vi "EXAMPLE64.VI"() -> ()   [LabVIEW 2014]
uses:
  wlcomp.dll
  C:/Program Files (x86)/LCard/LIBRARY/BIN/wlcomp64.dll
panel:
  out "Numeric":i32
  out "Краткое описание":string="Данный пример поддерживает платы L761 L780 L783 L791 и модули E-154 E14-140 E14-440 E20-10. В примере осуществляется сбор 8192 отсчетов с 4 каналов АЦП на максимальной скорости (для E20-10 на скорости 1МГц). Перед началом работы необходимо ввести имя фала с биос для платы (без расширения, для модулей без биоса произвольно) и номер слота, где установлена плата. См. также файд instruct.html."
  out "TTL Input (IoAsync demo)":i32
  in  "SynchroType\n3 - without sync(L7XX E2010)\n0 - without sync(E440 E140 E154 L791)":u32=3
  in  "Enter slot number":u32
  in  "Enter bios name":string="l761"
  out "Display":i16[][](graph)
  out "sync counter":u32
  in  "stop":bool
  out "data addr":u32
  out "sync addr":u32
  out "size":u32
  out "dRate":dbl format="%.2f"
  out "FIFO":u32
  out "IrqStep":u32
  out "Pages":u32
  out "Alloc":u32
  out "Error":u32
  out "IsDacPresent":u16
  out "Quartz":i32
  out "DspType":string
  out "Rev":string
  out "BrdName":string
  out "SerNum":string
  out "Base I/O":u32 format="%.0x"
  out "Irq":u32
  out "Dsp":u32
  out "BoardType":u32
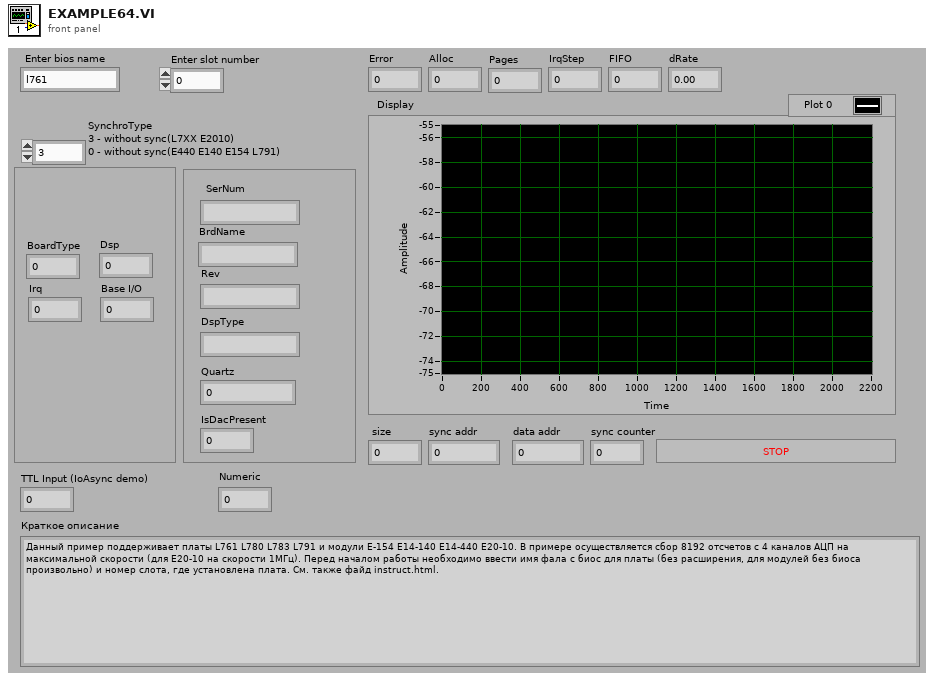
[diagram p1: front panel]
types:
  T1 = cluster{"s_Type":u32, "FIFO":u32, "IrqStep":u32, "Pages":u32, "Autoinit":u32, "dRate":dbl, "dKadr":dbl, "dScale":dbl, "Rate":u32, "Kadr":u32, "Scale":u32, "FPDelay":u32, "SynchroType\n3 - without sync(L7XX E2010)\n0 - without sync(E440 E140 E154 L791)":u32, "SynchroSensitivity":u32, "SynchroMode":u32, "AdChannel":u32, "AdPorog":u32, "NCh":u32, u32[], "IrqEna":u32, "AdcEna":u32}
  T2 = cluster{"[0]":u32, "[1]":u32, "[2]":u32, "[3]":u32, "[4]":u32, "[5]":u32, "[6]":u32, "[7]":u32, "[8]":u32, "[9]":u32, "[10]":u32, "[11]":u32, "[12]":u32, "[13]":u32, "[14]":u32, "[15]":u32, "[16]":u32, "[17]":u32, "[18]":u32, "[19]":u32}
  T3 = cluster{string, string, string, string, i32, u16}
  T4 = cluster{"s_Type":u32, "FIFO":u32, "IrqStep":u32, "Pages":u32, "dRate":dbl, "Rate":u32, "NCh":u32, "Chn[0]":u32, "Data[0]":u32, "Chn[1]":u32, "Data[1]":u32, "Mode":u32}
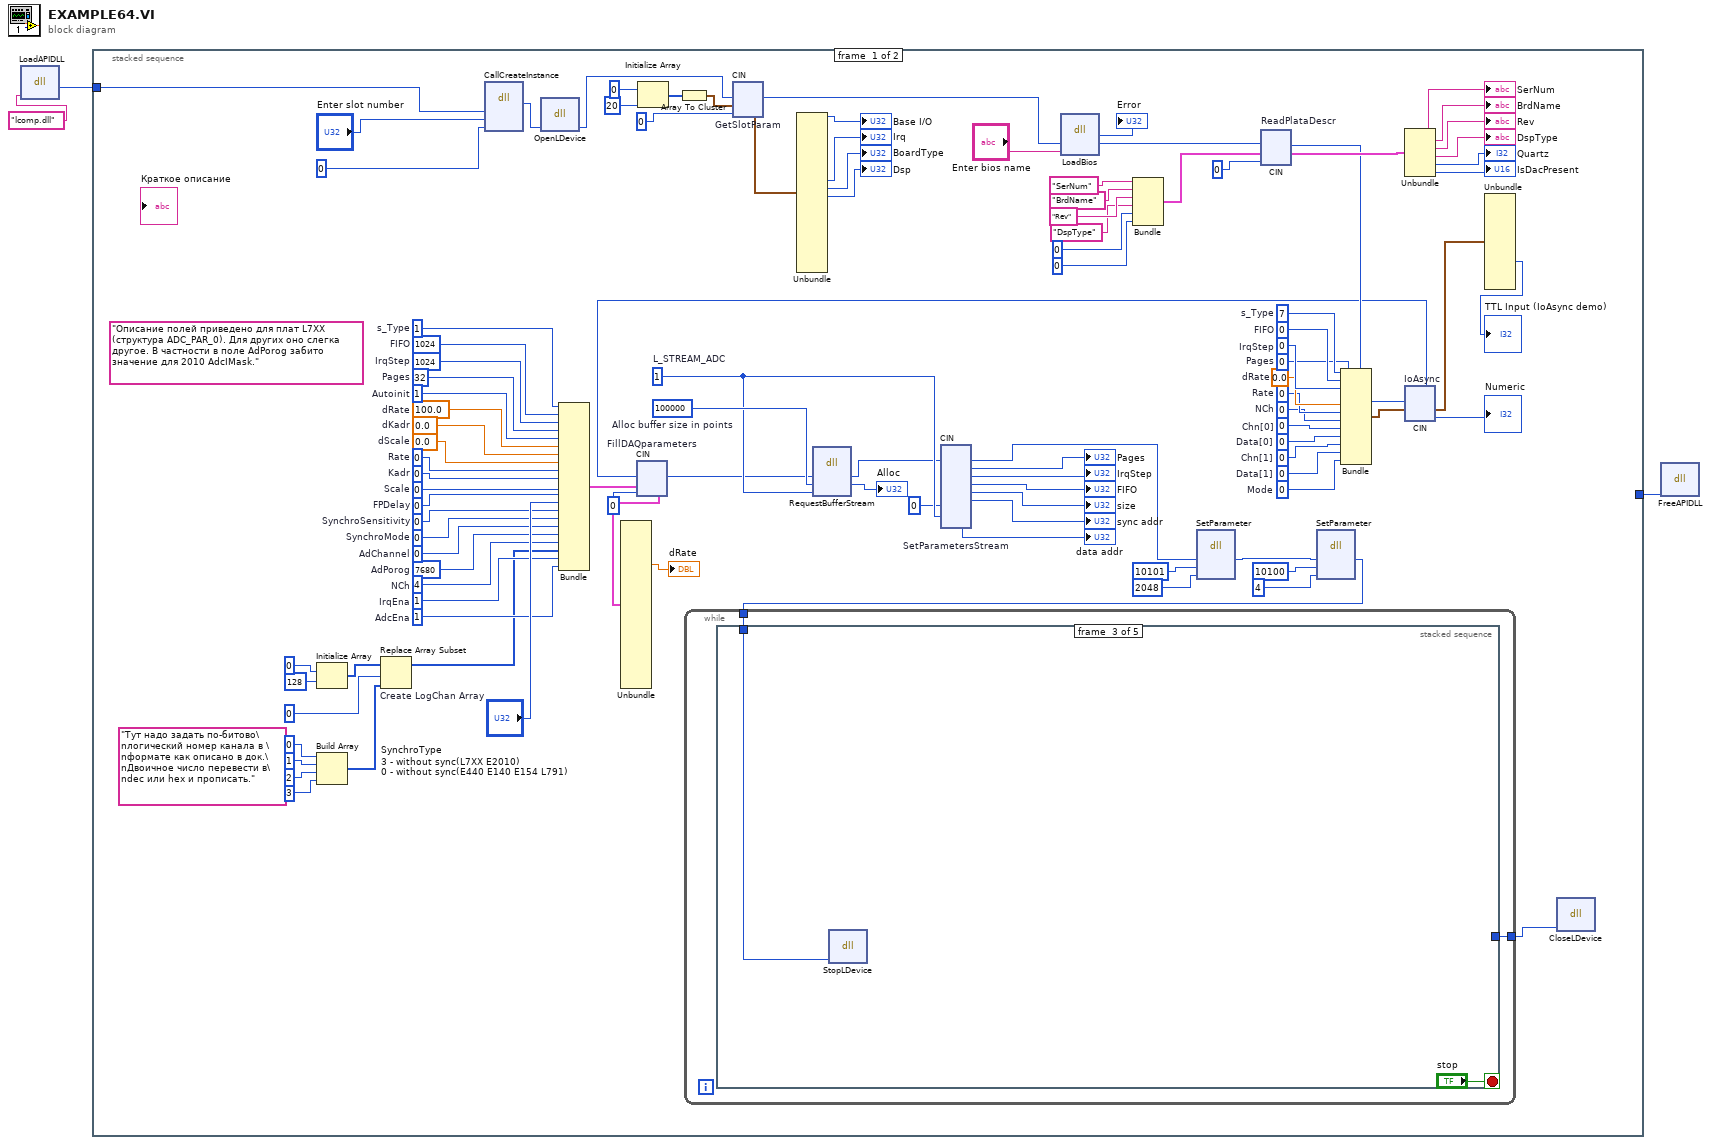
[diagram p0: block diagram]
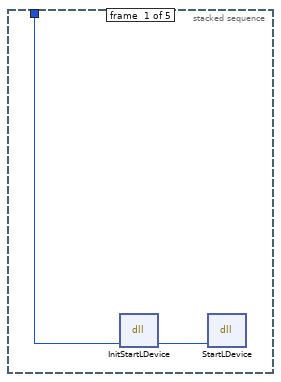
[diagram p2: hidden frame]
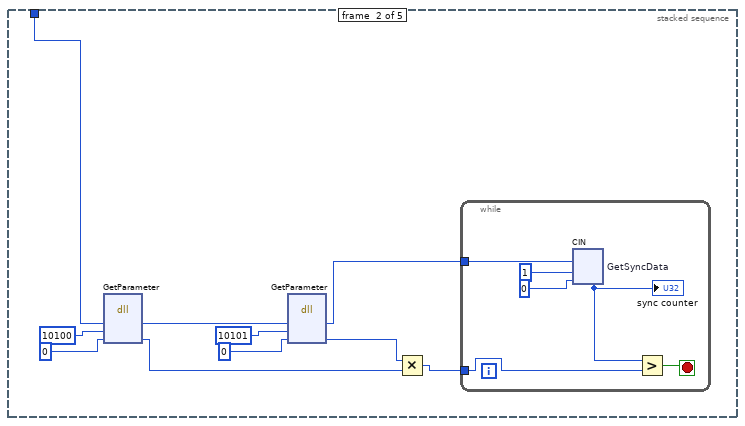
[diagram p3: hidden frame]
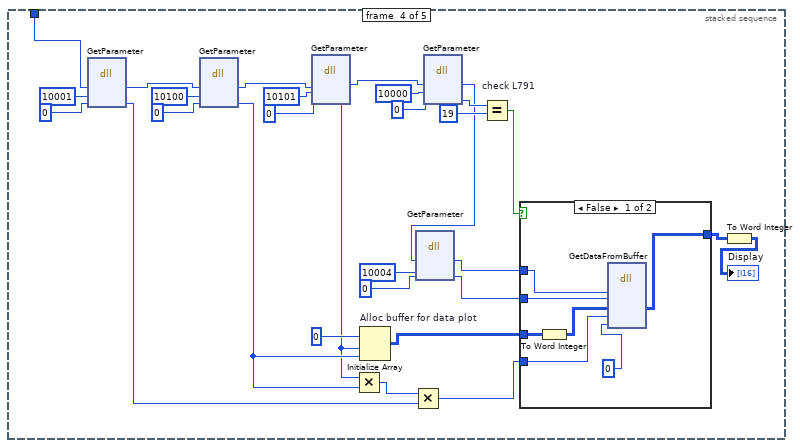
[diagram p4: hidden frame]
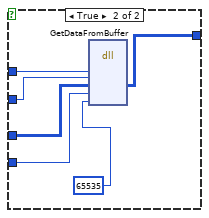
[diagram p5: hidden frame]
diagram:
  n1 = dll-call lib="wlcomp.dll" fn="LoadAPIDLL" label="LoadAPIDll"("dllname"="lcomp.dll") -> (w1:u32)  [unwired: 4 in, 2 out]
  n2 = stacked-sequence {
    tunnel: w1 -> [w105 w175]
    tunnel: [_ w175] -> w2
    frame #0 {
      w4 = u32 0  # Data[1]
      w5 = u32 0  # Chn[1]
      (unwired) "Тут надо задать по-битово\nлогический номер канала в \nформате как описано в док.\nДвоичное число перевести в\ndec или hex и прописать."
      (unwired) "Описание полей приведено для плат L7XX (структура ADC_PAR_0). Для других оно слегка другое. В частности в поле AdPorog забито значение для 2010 AdcIMask."
      w32 = u32 0  # Mode
      w23 = u32 0  # Data[0]
      w24 = u32 0  # Chn[0]
      w25 = u32 0  # NCh
      w26 = u32 0  # Rate
      w27 = 0.0  # dRate
      w28 = u32 0  # Pages
      w29 = u32 0  # IrqStep
      w30 = u32 0  # FIFO
      w31 = u32 7  # s_Type
      w52 = u32 1  # L_STREAM_ADC
      w53 = u32 100000  # Alloc buffer size in points
      w64 = u32 1  # AdcEna
      w65 = u32 1  # IrqEna
      w66 = u32 4  # NCh
      w67 = u32 7680  # AdPorog
      w68 = u32 0  # AdChannel
      w69 = u32 0  # SynchroMode
      w70 = u32 0  # SynchroSensitivity
      w72 = u32 0  # FPDelay
      w73 = u32 0  # Scale
      w74 = u32 0  # Kadr
      w75 = u32 0  # Rate
      w76 = 0.0  # dScale
      w77 = 0.0  # dKadr
      w78 = 100.0  # dRate
      w79 = u32 1  # Autoinit
      w80 = u32 32  # Pages
      w81 = u32 1024  # IrqStep
      w82 = u32 1024  # FIFO
      w83 = u32 1  # s_Type
      n3 = Initialize Array(u32 0, u32 128) -> (w61:u32[])
      n4 = Build Array(0, 1, 2, 3) -> (w58:i32[])
      n5 = Replace Array Subset "Create LogChan Array"(array=w61, new element=w58, index=u32 0) -> (w60:u32[])
      n6 = dll-call lib="wlcomp.dll" fn="CallCreateInstance"("hDll"=w105, "slot"="Enter slot number", "Err"=u32 0) -> (w46:u32)  [unwired: 6 in, 2 out]
      n7 = dll-call lib="wlcomp.dll" fn="OpenLDevice"("hIfc"=w46) -> ("hIfc"=w45:u32)  [unwired: 4 in, 2 out]
      n8 = Bundle("s_Type"=w83, "FIFO"=w82, "IrqStep"=w81, "Pages"=w80, "Autoinit"=w79, "dRate"=w78, "dKadr"=w77, "dScale"=w76, "Rate"=w75, "Kadr"=w74, "Scale"=w73, "FPDelay"=w72, "SynchroType\n3 - without sync(L7XX E2010)\n0 - without sync(E440 E140 E154 L791)"="SynchroType\n3 - without sync(L7XX E2010)\n0 - without sync(E440 E140 E154 L791)", "SynchroSensitivity"=w70, "SynchroMode"=w69, "AdChannel"=w68, "AdPorog"=w67, "NCh"=w66, w60, "IrqEna"=w65, "AdcEna"=w64) -> (w84:T1)  [unwired: 1 in]
      n9 = Initialize Array(u32 0, u32 20) -> (w107:u32[])
      n10 = Array To Cluster(array=w107) -> (cluster=w99:T2)
      n11 = cin "GetSlotParam"(w45, w99, u32 0) -> (w39:u32, w98:T2)  [unwired: 1 in]
      n12 = Unbundle(w98) -> ("[0]"=→"Base I/O":u32, "[8]"=→"Irq":u32, "[9]"=→"BoardType":u32, "[10]"=→"Dsp":u32)  [unwired: 16 out]
      n13 = dll-call lib="wlcomp.dll" fn="LoadBios"("hIfc"=w39, "BiosName"="Enter bios name") -> (→"Error":u32, "hIfc"=w38:u32)  [unwired: 4 in, 2 out]
      n14 = Bundle("SerNum", "BrdName", "Rev", "DspType", 0, u16 0) -> (w35:T3)  [unwired: 1 in]
      n15 = cin "ReadPlataDescr"(w38, w35, u32 0) -> (w17:u32, w91:T3)  [unwired: 1 in]
      n16 = Bundle("s_Type"=w31, "FIFO"=w30, "IrqStep"=w29, "Pages"=w28, "dRate"=w27, "Rate"=w26, "NCh"=w25, "Chn[0]"=w24, "Data[0]"=w23, "Chn[1]"=w5, "Data[1]"=w4, "Mode"=w32) -> (w22:T4)  [unwired: 1 in]
      n17 = Unbundle(w91) -> (→"SerNum":string, →"BrdName":string, →"Rev":string, →"DspType":string, →"Quartz":i32, →"IsDacPresent":u16)
      n18 = cin "IoAsync"(w17, w22) -> (w16:u32, w21:T4, →"Numeric":i32)  [unwired: 1 in]
      n19 = cin "FillDAQparameters"(w16, w84, 0) -> (w42:u32, w34:T1)  [unwired: 1 in]
      n20 = Unbundle(w34) -> ("dRate"=→"dRate":dbl)  [unwired: 20 out]
      n21 = dll-call lib="wlcomp.dll" fn="RequestBufferStream" label="RequestBuffer"("hIfc"=w42, "Size"=w53, "StreamId"=w52) -> ("hIfc"=w41:u32, "Size"=→"Alloc":u32)  [unwired: 5 in, 2 out]
      n22 = cin "SetParametersStream"(w41, w52, u32 0) -> (w10:u32, →"Pages":u32, →"IrqStep":u32, →"FIFO":u32, →"size":u32, →"sync addr":u32, →"data addr":u32)  [unwired: 8 in]
      n23 = dll-call lib="wlcomp.dll" fn="SetParameter" label="Store point per chan"("hIfc"=w10, "name"=10101, "param"=2048) -> ("hIfc"=w6:u32)  [unwired: 6 in, 2 out]
      n24 = dll-call lib="wlcomp.dll" fn="SetParameter" label="Store NCh"("hIfc"=w6, "name"=10100, "param"=4) -> ("hIfc"=w7:u32)  [unwired: 6 in, 2 out]
      n25 = while {
        tunnel: w7 -> [w111]
        tunnel: [w110] -> w13
        stop <- "stop" stop-if-true
        n26 = stacked-sequence {
          tunnel: w111 -> [w113 w116 w131 w147 w174]
          tunnel: [_ _ _ _ w174] -> w110
          frame #0 {
            n27 = dll-call lib="wlcomp.dll" fn="InitStartLDevice"("hIfc"=w113) -> ("hIfc"=w114:u32)  [unwired: 4 in, 2 out]
            n28 = dll-call lib="wlcomp.dll" fn="StartLDevice"("hIfc"=w114) -> ()  [unwired: 5 in, 2 out]
          }
          frame #1 {
            n29 = dll-call lib="wlcomp.dll" fn="GetParameter" label="Get NCh"("hIfc"=w116, "name"=10100, "param"=0) -> ("hIfc"=w121:u32, "param"=w123:u32)  [unwired: 5 in, 2 out]
            n30 = dll-call lib="wlcomp.dll" fn="GetParameter" label="Get points per chan"("hIfc"=w121, "name"=10101, "param"=0) -> ("hIfc"=w115:u32, "param"=w122:u32)  [unwired: 5 in, 2 out]
            n31 = Multiply(x=w122, y=w123) -> (x*y=w124:u32)
            n32 = while {
              tunnel: w115 -> [w126]
              tunnel: w124 -> [w125]
              stop <- w130 stop-if-true
              n33 = cin "GetSyncData"(w126, 1, u32 0) -> (w127:u32)  [unwired: 2 in]
              "sync counter" <- w127
              n34 = Greater?(x=w127, y=w125) -> (0:w130:bool)
            }
          }
          frame #2 {
            n35 = dll-call lib="wlcomp.dll" fn="StopLDevice"("hIfc"=w131) -> ()  [unwired: 5 in, 2 out]
          }
          frame #3 {
            n36 = dll-call lib="wlcomp.dll" fn="GetParameter" label="Get DataPoint size"("hIfc"=w147, "name"=10001, "param"=0) -> ("hIfc"=w134:u32, "param"=w151:u32)  [unwired: 5 in, 2 out]
            n37 = dll-call lib="wlcomp.dll" fn="GetParameter" label="Get NCh"("hIfc"=w134, "name"=10100, "param"=0) -> ("hIfc"=w135:u32, "param"=w133:u32)  [unwired: 5 in, 2 out]
            n38 = dll-call lib="wlcomp.dll" fn="GetParameter" label="Get points per chan"("hIfc"=w135, "name"=10101, "param"=0) -> ("hIfc"=w138:u32, "param"=w132:u32)  [unwired: 5 in, 2 out]
            n39 = Multiply(x=w132, y=w133) -> (x*y=w146:u32)
            n40 = Initialize Array "Alloc buffer for data plot"(u32 0, w132, w133) -> (w154:u32[][])
            n41 = Multiply(x=w146, y=w151) -> (x*y=w156:u32)
            n42 = dll-call lib="wlcomp.dll" fn="GetParameter" label="Get BoardType"("hIfc"=w138, "name"=10000, "param"=0) -> ("hIfc"=w143:u32, "param"=w148:u32)  [unwired: 5 in, 2 out]
            n43 = dll-call lib="wlcomp.dll" fn="GetParameter" label="Get DataAddr"("hIfc"=w143, "name"=10004, "param"=0) -> ("hIfc"=w142:u32, "param"=w141:u32)  [unwired: 5 in, 2 out]
            n44 = Equal? "check L791"(x=w148, y=19) -> (x = y?=w159:bool)
            n45 = case shown="False" w159 {
              tunnel: [w167 w173] -> w158
              tunnel: w142 -> [w166 w172]
              tunnel: w141 -> [w165 w171]
              tunnel: w154 -> [w163 w170]
              tunnel: w156 -> [w164 w169]
              frame False {
                n46 = To Word Integer(number=w163) -> (16bit integer=w162:i16[][])
                n47 = dll-call lib="wlcomp.dll" fn="GetDataFromBuffer"("hIfc"=w166, "data"=w165, "datad"=w162, "size"=w164, "mask"=u32 0) -> ("datad"=w167:i16[][])  [unwired: 8 in, 2 out]
              }
              frame True {
                n48 = dll-call lib="wlcomp.dll" fn="GetDataFromBuffer"("hIfc"=w172, "data"=w171, "datad"=w170, "size"=w169, "mask"=65535) -> ("datad"=w173:u32[][])  [unwired: 8 in, 2 out]
              }
            }
            n49 = To Word Integer(number=w158) -> (16bit integer=→"Display":i16[][])
          }
          frame #4 {
          }
        }
      }
      n50 = Unbundle(w21) -> ("Data[0]"=→"TTL Input (IoAsync demo)":u32)  [unwired: 11 out]
      n51 = dll-call lib="wlcomp.dll" fn="CloseLDevice"("hIfc"=w13) -> ()  [unwired: 5 in, 2 out]
    }
    frame #1 {
    }
  }
  n52 = dll-call lib="C:/Program Files (x86)/LCard/LIBRARY/BIN/wlcomp64.dll" fn="FreeAPIDLL" label="FreeAPIDll"("hDll"=w2) -> ()  [unwired: 5 in, 2 out]
